vi "ReadVXM-subsyLookup.vi"(8 "error in":errorcluster, 11 "Motion Cfg File path":path=path "C:/Users/Public/Documents/OU PAARD/mmWave_RF_Scanner/SupportFiles/VXMtoSubsysLookup.csv") -> (0 "error out":errorcluster, 3 "Lookup Table":T1(array[cluster]))   [LabVIEW 2017]
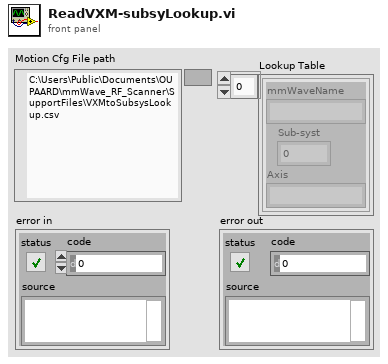
[diagram p1: front panel]
types:
  T1 = cluster{"mmWaveName":string, "Sub-syst":i32, "Axis":string}[]
  T2 = cluster{"mmWaveName":string, "Sub-syst":i32, "Axis":string}
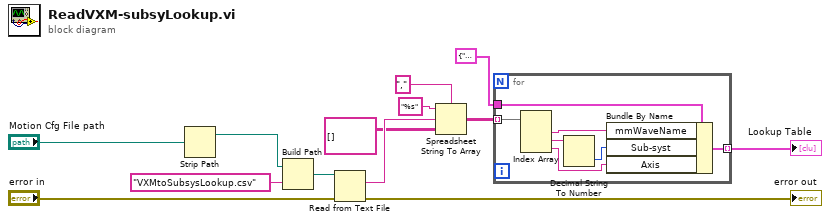
[diagram p0: block diagram]
diagram:
  n1 = Strip Path(path="Motion Cfg File path") -> (stripped path=w13:path)  [unwired: 1 out]
  n2 = Build Path(base path=w13, name or relative path="VXMtoSubsysLookup.csv") -> (appended path=w10:path)
  n3 = Read from Text File(file (use dialog)=w10, error in="error in") -> (text=w9:string, error out=→"error out":errorcluster)  [unwired: 2 in, 2 out]
  n4 = Spreadsheet String To Array(delimiter (Tab)=",", format string="%s", spreadsheet string=w9, array type (2D Dbl)=string[][] []) -> (array=w5:string[][])
  n5 = for {
    tunnel: w5 -> [w20] mode=indexing
    tunnel: [w15] -> w3 mode=indexing
    tunnel: T2 {"mmWaveName"="", "Sub-syst"=0, "Axis"=""} ("output cluster") -> [w14]
    n6 = Index Array(array=w20) -> (element #1=w17:string, element #2=w19:string, element #3=w16:string)  [unwired: 3 in]
    n7 = Decimal String To Number(string=w19) -> (number=w18:i32)  [unwired: 2 in, 1 out]
    n8 = Bundle By Name(cluster=w14, "mmWaveName"=w17, "Sub-syst"=w18, "Axis"=w16) -> (w15:T2)
  }
  "Lookup Table" <- w3
